vi "string_nodes.vi"() -> ()   [LabVIEW 2023]
panel:
  out "Waveform Graph":cluster{i32, dbl, dbl[]}(graph)
  in  "Slide":i32(slide) scale=0.0..10.0
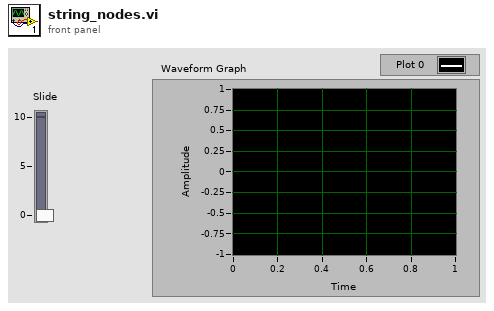
[diagram p1: front panel]
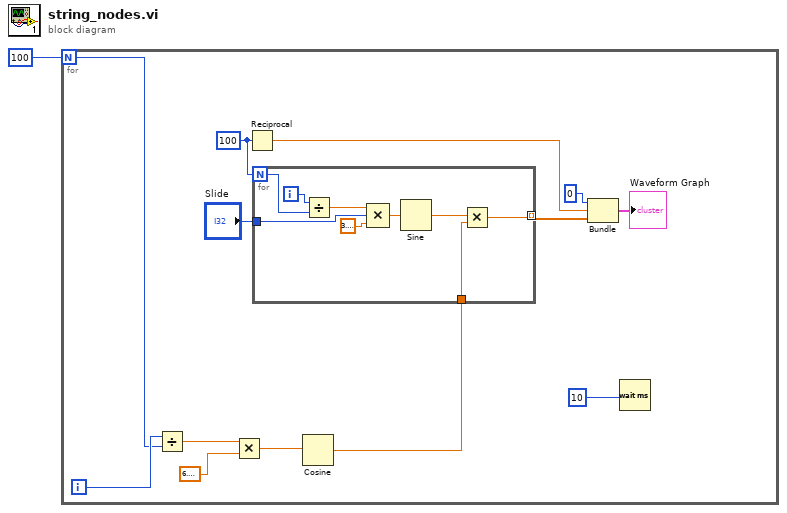
[diagram p0: block diagram]
diagram:
  n1 = for {
    N: 100 -> [w7]
    i -> [w8]
    w13 = 100
    n2 = Divide(x=w8, y=w7) -> (x/y=w6:dbl)
    n3 = Multiply(x=w6, y=6.283185307179586) -> (x*y=w4:dbl)
    n4 = Reciprocal(x=w13) -> (1/x=w12:dbl)
    n5 = Cosine(x=w4) -> (cos(x)=w3:dbl)
    n6 = for {
      N: w13 -> [w22]
      tunnel: [w15] -> w14 mode=indexing
      tunnel: "Slide" -> [w18]
      tunnel: w3 -> [w16]
      i -> [w23]
      n7 = Divide(x=w23, y=w22) -> (x/y=w21:dbl)
      n8 = Compound Arithmetic op=MULTIPLY(w21, w18, 3.141592653589793) -> (w19:dbl)
      n9 = Sine(x=w19) -> (sin(x)=w17:dbl)
      n10 = Multiply(x=w17, y=w16) -> (x*y=w15:dbl)
    }
    n11 = Bundle(0, w12, w14) -> (→"Waveform Graph":cluster{i32, dbl, dbl[]})  [unwired: 1 in]
    n12 = Wait (ms)(milliseconds to wait=10) -> ()  [unwired: 1 out]
  }
